vi "Append First Packet.vi"(6 "Repeat Scan":i32, 7 "MAC Address":string, 8 "Ny":i32, 9 "Nx":i32, 10 "Packets":string[](array[string]), 11 "AOL_Globals":T1={"Imaging Protocol"=enum."AOL Z-Stack", "Number of POI"=0, "Number of Miniscans"=0, "Number of Trials"=0, "Number of Cycles "=0, "# Averaged Frames"=0, "Laser power (%)"=0, "Pockels"=0.0, "Acquisition Length (sec)"=0.0, "Fill time (us)"=0.0, "POI Dwell time (us)"=0.0, "Miniscan Dwell time per pixel (us)"=0.0, "PMT 1"=0.0, "PMT 2"=0.0, "Back Apperture"=0.0, "Frame Size"=0, "Center Frequency"=0.0, "Field of View"=0.0, "DwellTime (us)"=0.0, "Wavelength (nm)"=0.0, "Zoom"=0.0, "AOL Z"=0.0, "AOL Mode"=enum."Raster", "GridXY"=0.0, "GridZ"=0.0, "TriggerPeriod (sec)"=0.0, "Number of Pixels in Miniscan"=0, "Experiment folder path"=path "", "X centre"=0.0, "Y centre"=0.0, "Angle (degrees)"=0.0, "Plane Mode"=0, "Threshold"=[], "Regenerate Chirps"=FALSE, "Rectangle ROI length (pixels)"=0, "Rectangle ROI height (pixels)"=0, "AOD fill"=0, "Samples Wait after Trigger"=0, "StartUp Delay"=0, "Slip Cycle"=163840, "Add Cycle"=FALSE} {"Plane Mode" items=["XY Plane"]; "Frame Size" items=["100X100"=100, "128X128"=128, "200X200"=200, "256X256"=256, "512X512"=512, "1024x1024"=1024, "2048x2048"=2048]; "Back Apperture" format="%#.6g"; "Pockels" format="%#.6g"; "PMT 2" format="%#.6g"; "PMT 1" format="%#.6g"; "Angle (degrees)" format="%#.6g"; "POI Dwell time (us)" format="%#.6g"}) -> (0 "Repeat":i32, 2 "HexPackets":string[](array[string]), 3 "Total Packets":i32)   [LabVIEW 2013]
uses:
  Typedefs/Controls/AOL_Globals.ctl
  Typedefs/Imaging Protocols enum.ctl
  Typedefs/Frame Size.ctl
  Typedefs/AOL modes.ctl
  Typedefs/Plane Mode.ctl
panel:
  # "RE-ENTRANT"
  # "SUB-ROUTINE"
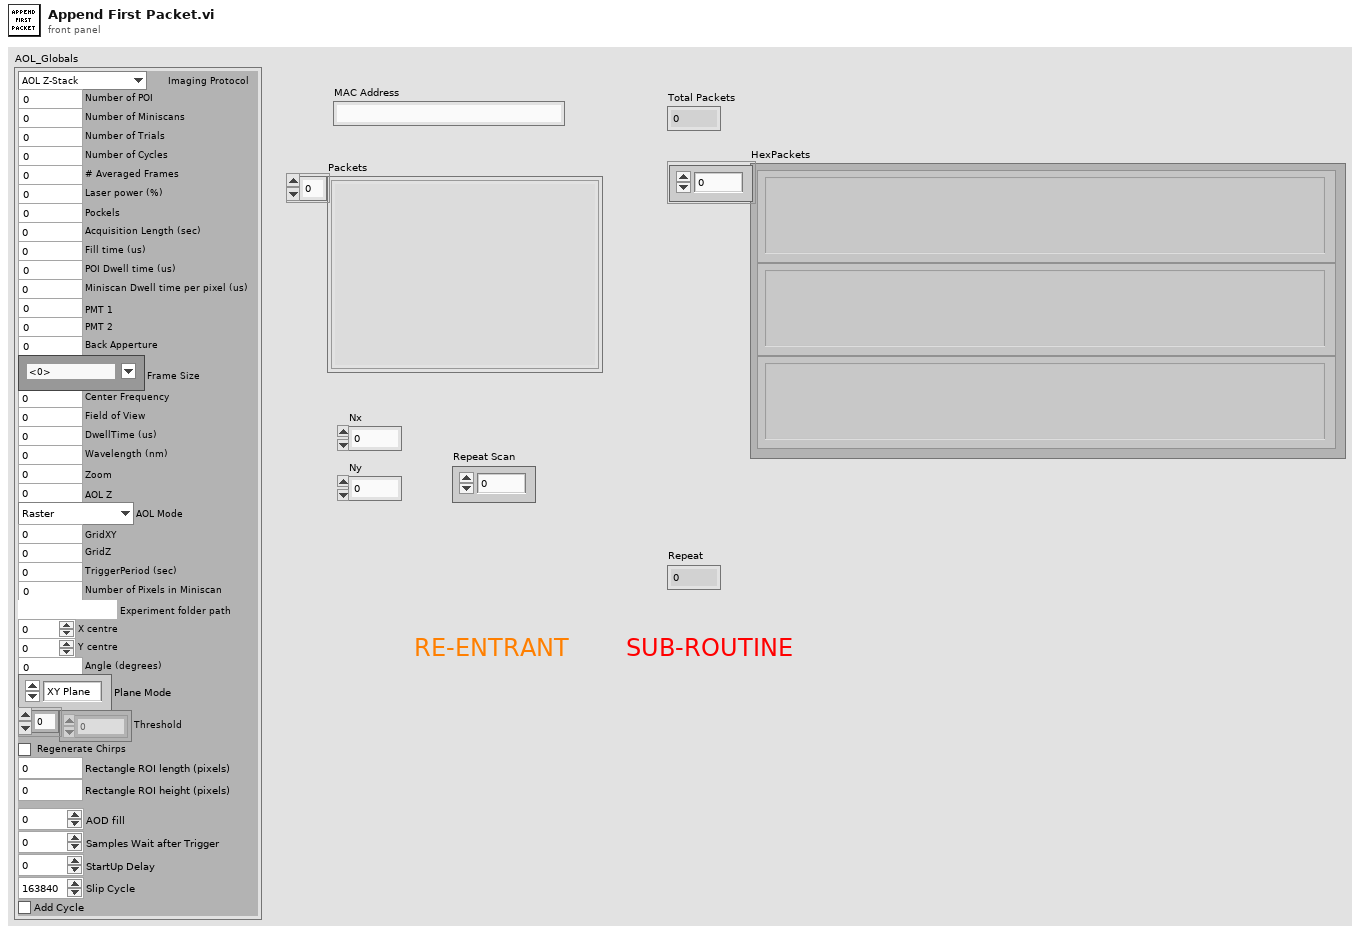
[diagram p1: front panel]
types:
  T1 = typedef "AOL_Globals.ctl" = cluster{"Imaging Protocol":T2, "Number of POI":u16, "Number of Miniscans":u16, "Number of Trials":u16, "Number of Cycles ":u64, "# Averaged Frames":u16, "Laser power (%)":u8, "Pockels":dbl, "Acquisition Length (sec)":dbl, "Fill time (us)":dbl, "POI Dwell time (us)":dbl, "Miniscan Dwell time per pixel (us)":dbl, "PMT 1":dbl, "PMT 2":dbl, "Back Apperture":dbl, "Frame Size":T3, "Center Frequency":dbl, "Field of View":dbl, "DwellTime (us)":dbl, "Wavelength (nm)":dbl, "Zoom":dbl, "AOL Z":dbl, "AOL Mode":T4, "GridXY":dbl, "GridZ":dbl, "TriggerPeriod (sec)":dbl, "Number of Pixels in Miniscan":u16, "Experiment folder path":path, "X centre":dbl, "Y centre":dbl, "Angle (degrees)":dbl, "Plane Mode":T5, "Threshold":u16[], "Regenerate Chirps":bool, "Rectangle ROI length (pixels)":u16, "Rectangle ROI height (pixels)":u16, "AOD fill":u16, "Samples Wait after Trigger":u16, "StartUp Delay":i32, "Slip Cycle":u32, "Add Cycle":bool}
  T2 = typedef "Imaging Protocols enum.ctl" = enum16{"AOL Z-Stack", "Motor Z Stack", "Functional Acquisition", "Single Plane Acquisition", "Volume Acquisition", "Live Imaging", "Live Plane Imaging", "Live Volume Imaging"}
  T3 = typedef "Frame Size.ctl" = u16
  T4 = typedef "AOL modes.ctl" = enum16{"Raster", "Structural", "Pointing", "Mini Scan", "Alignment"}
  T5 = typedef "Plane Mode.ctl" = u16
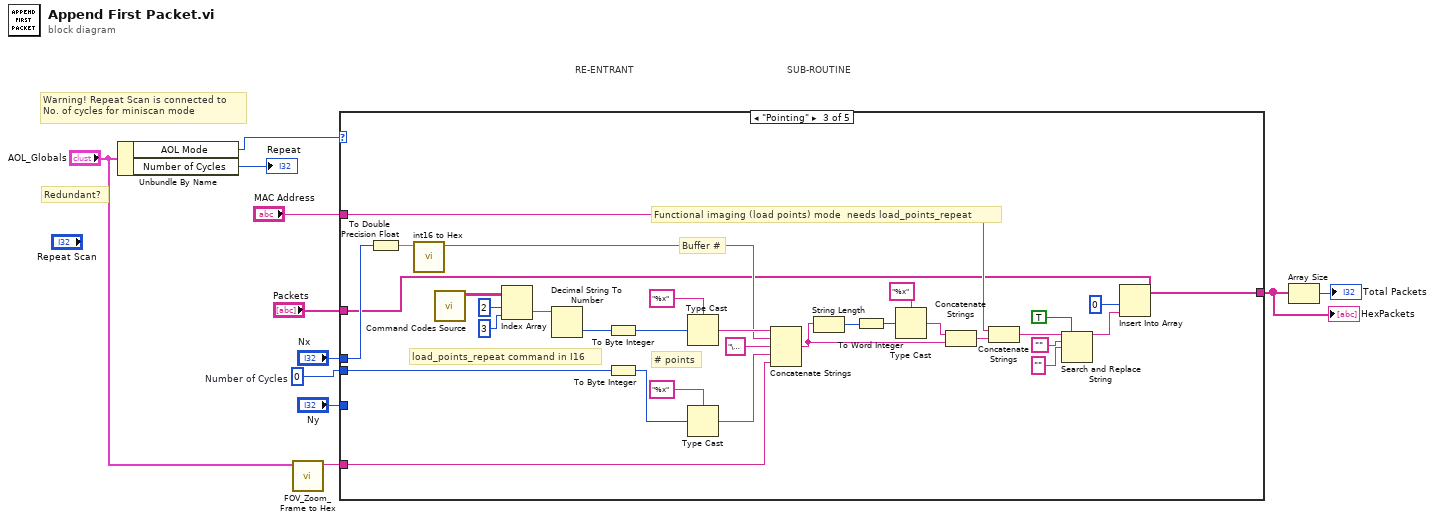
[diagram p0: block diagram]
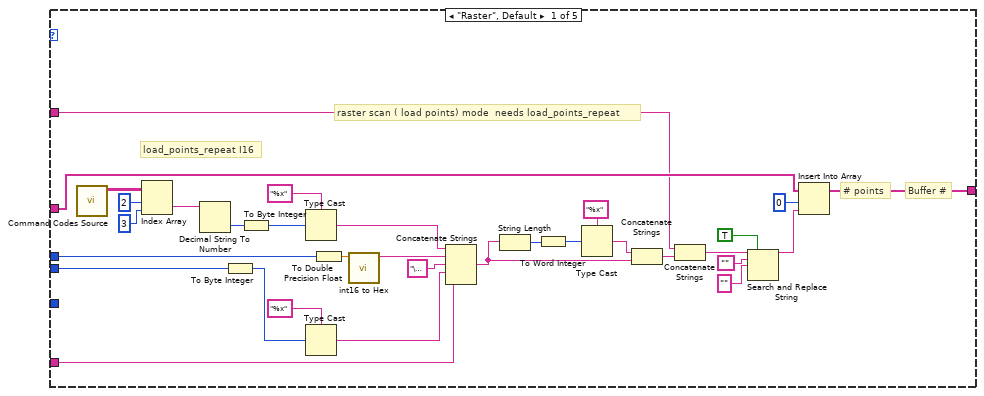
[diagram p2: hidden frame]
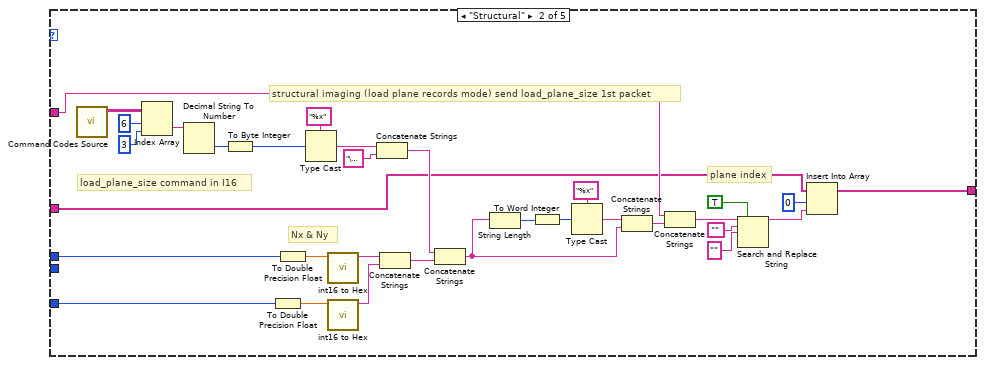
[diagram p3: hidden frame]
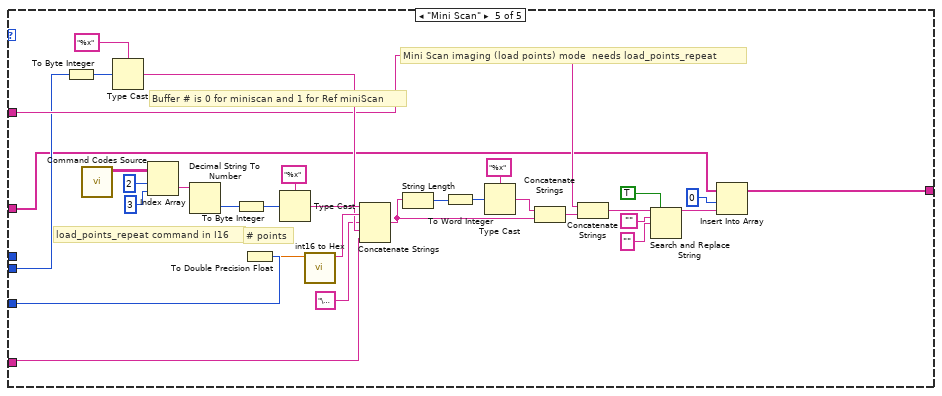
[diagram p5: hidden frame]
diagram:
  w3 = u16 0  # Number of Cycles
  # "SUB-ROUTINE"
  # "RE-ENTRANT"
  # "Redundant?"
  # "Warning! Repeat Scan is connected to \nNo. of cycles for miniscan mode"
  n1 = Unbundle By Name("AOL_Globals") -> ("AOL Mode"=w8:T4, "Number of Cycles"=→"Repeat":u64)
  n2 = call "FOV_Zoom_Frame to Hex.vi"("AOL_Globals"="AOL_Globals") -> ("FOV-Zoom-FrameSize Hex"=w1:string)  [unwired: 10 in]
  n3 = case shown="\"Pointing\"" w8 {
    tunnel: [w20 w48 w84 w108 w116] -> w9
    tunnel: "Ny" -> [_ w52 _ _ w114]
    tunnel: "Nx" -> [w25 w51 w89 _ _]
    tunnel: w3 -> [w15 _ w83 _ w113]
    tunnel: "Packets" -> [w22 w44 w76 w108 w110]
    tunnel: "MAC Address" -> [w16 w47 w79 _ w115]
    tunnel: w1 -> [w13 _ w77 _ w111]
    frame "Raster", Default {
      # "load_points_repeat I16"
      # "# points"
      # "Buffer #"
      # "raster scan ( load points) mode  needs load_points_repeat"
      n4 = call "Command Codes Source.vi"() -> ("Commands for FPGA"=w34:string[][])  [unwired: 11 in]
      n5 = Index Array(array=w34, index (row)=2 ("disabled index (row)"), index (col)=3 ("disabled index (col)")) -> (element=w28:string)
      n6 = Decimal String To Number(string=w28) -> (number=w30:i32)  [unwired: 2 in, 1 out]
      n7 = To Byte Integer(number=w15) -> (8bit integer=w18:i8)
      n8 = To Byte Integer(number=w30) -> (8bit integer=w29:i8)
      n9 = Type Cast(type="%x", x=w29) -> (*(type *) &x=w27:string)
      n10 = Type Cast(type="%x", x=w18) -> (*(type *) &x=w17:string)
      n11 = To Double Precision Float(number=w25) -> (double precision float=w14:dbl)
      n12 = call "int16 to Hex.vi"("number"=w14) -> ("Hex string"=w24:string)  [unwired: 10 in]
      n13 = Concatenate Strings(w27, w24, "\u0000" ("string"), w17, w13) -> (w26:string)
      n14 = String Length(string=w26) -> (length=w40:i32)
      n15 = To Word Integer(number=w40) -> (16bit integer=w35:i16)
      n16 = Type Cast(type="%x", x=w35) -> (*(type *) &x=w42:string)
      n17 = Concatenate Strings(w42, w26) -> (w43:string)
      n18 = Concatenate Strings(w16, w43) -> (w39:string)
      n19 = Search and Replace String(replace all?=TRUE ("replace all? (F)"), input string=w39, search string="", replace string="" ("replace string (\"\")")) -> (result string=w21:string)  [unwired: 4 in, 3 out]
      n20 = Insert Into Array(array=w22, index=0, new element=w21) -> (w20:string[])
    }
    frame "Structural" {
      # "load_plane_size command in I16"
      # "Nx & Ny"
      # "plane index"
      # "structural imaging (load plane records mode) send load_plane_size 1st packet"
      n21 = call "Command Codes Source.vi"() -> ("Commands for FPGA"=w66:string[][])  [unwired: 11 in]
      n22 = Index Array(array=w66, index (row)=6 ("disabled index (row)"), index (col)=3 ("disabled index (col)")) -> (element=w60:string)
      n23 = Decimal String To Number(string=w60) -> (number=w62:i32)  [unwired: 2 in, 1 out]
      n24 = To Byte Integer(number=w62) -> (8bit integer=w61:i8)
      n25 = To Double Precision Float(number=w52) -> (double precision float=w45:dbl)
      n26 = To Double Precision Float(number=w51) -> (double precision float=w46:dbl)
      n27 = Type Cast(type="%x", x=w61) -> (*(type *) &x=w59:string)
      n28 = call "int16 to Hex.vi"("number"=w46) -> ("Hex string"=w56:string)  [unwired: 10 in]
      n29 = call "int16 to Hex.vi"("number"=w45) -> ("Hex string"=w55:string)  [unwired: 10 in]
      n30 = Concatenate Strings(w59, "\u0000" ("string")) -> (w57:string)
      n31 = Concatenate Strings(w56, w55) -> (w54:string)
      n32 = Concatenate Strings(w57, w54) -> (w53:string)
      n33 = String Length(string=w53) -> (length=w72:i32)
      n34 = To Word Integer(number=w72) -> (16bit integer=w67:i16)
      n35 = Type Cast(type="%x", x=w67) -> (*(type *) &x=w74:string)
      n36 = Concatenate Strings(w74, w53) -> (w75:string)
      n37 = Concatenate Strings(w47, w75) -> (w71:string)
      n38 = Search and Replace String(replace all?=TRUE ("replace all? (F)"), input string=w71, search string="", replace string="" ("replace string (\"\")")) -> (result string=w49:string)  [unwired: 4 in, 3 out]
      n39 = Insert Into Array(array=w44, index=0, new element=w49) -> (w48:string[])
    }
    frame "Pointing" {
      # "load_points_repeat command in I16"
      # "# points"
      # "Buffer #"
      # "Functional imaging (load points) mode  needs load_points_repeat"
      n40 = To Double Precision Float(number=w89) -> (double precision float=w78:dbl)
      n41 = call "int16 to Hex.vi"("number"=w78) -> ("Hex string"=w88:string)  [unwired: 10 in]
      n42 = call "Command Codes Source.vi"() -> ("Commands for FPGA"=w98:string[][])  [unwired: 11 in]
      n43 = Index Array(array=w98, index (row)=2 ("disabled index (row)"), index (col)=3 ("disabled index (col)")) -> (element=w92:string)
      n44 = Decimal String To Number(string=w92) -> (number=w94:i32)  [unwired: 2 in, 1 out]
      n45 = To Byte Integer(number=w94) -> (8bit integer=w93:i8)
      n46 = To Byte Integer(number=w83) -> (8bit integer=w81:i8)
      n47 = Type Cast(type="%x", x=w93) -> (*(type *) &x=w91:string)
      n48 = Type Cast(type="%x", x=w81) -> (*(type *) &x=w80:string)
      n49 = Concatenate Strings(w91, w88, "\u0000" ("string"), w80, w77) -> (w90:string)
      n50 = String Length(string=w90) -> (length=w104:i32)
      n51 = To Word Integer(number=w104) -> (16bit integer=w99:i16)
      n52 = Type Cast(type="%x", x=w99) -> (*(type *) &x=w106:string)
      n53 = Concatenate Strings(w106, w90) -> (w107:string)
      n54 = Concatenate Strings(w79, w107) -> (w103:string)
      n55 = Search and Replace String(replace all?=TRUE ("replace all? (F)"), input string=w103, search string="", replace string="" ("replace string (\"\")")) -> (result string=w85:string)  [unwired: 4 in, 3 out]
      n56 = Insert Into Array(array=w76, index=0, new element=w85) -> (w84:string[])
    }
    frame "Alignment" {
      # "alignment mode is load single frquency"
    }
    frame "Mini Scan" {
      # "load_points_repeat command in I16"
      # "# points"
      # "Buffer # is 0 for miniscan and 1 for Ref miniScan"
      # "Mini Scan imaging (load points) mode  needs load_points_repeat"
      n57 = To Byte Integer(number=w113) -> (8bit integer=w118:i8)
      n58 = call "Command Codes Source.vi"() -> ("Commands for FPGA"=w131:string[][])  [unwired: 11 in]
      n59 = Type Cast(type="%x", x=w118) -> (*(type *) &x=w117:string)
      n60 = Index Array(array=w131, index (row)=2 ("disabled index (row)"), index (col)=3 ("disabled index (col)")) -> (element=w125:string)
      n61 = Decimal String To Number(string=w125) -> (number=w127:i32)  [unwired: 2 in, 1 out]
      n62 = To Byte Integer(number=w127) -> (8bit integer=w126:i8)
      n63 = To Double Precision Float(number=w114) -> (double precision float=w112:dbl)
      n64 = Type Cast(type="%x", x=w126) -> (*(type *) &x=w124:string)
      n65 = call "int16 to Hex.vi"("number"=w112) -> ("Hex string"=w122:string)  [unwired: 10 in]
      n66 = Concatenate Strings(w124, w122, "\u0000" ("string"), w117, w111) -> (w123:string)
      n67 = String Length(string=w123) -> (length=w137:i32)
      n68 = To Word Integer(number=w137) -> (16bit integer=w132:i16)
      n69 = Type Cast(type="%x", x=w132) -> (*(type *) &x=w139:string)
      n70 = Concatenate Strings(w139, w123) -> (w140:string)
      n71 = Concatenate Strings(w115, w140) -> (w136:string)
      n72 = Search and Replace String(replace all?=TRUE ("replace all? (F)"), input string=w136, search string="", replace string="" ("replace string (\"\")")) -> (result string=w120:string)  [unwired: 4 in, 3 out]
      n73 = Insert Into Array(array=w110, index=0, new element=w120) -> (w116:string[])
    }
  }
  "HexPackets" <- w9
  n74 = Array Size(array=w9) -> (size(s)=→"Total Packets":i32)
